vi "Check Home Position Part 2.vi"(8 "error in (no error)":errorcluster, 9 "Amphipods in":refnum<class "Amphipod.lvclass">[](array[class]), 10 "Home":i8, 11 "Position in":cluster{"Row":i8, "Column":i8}) -> (0 "error out":errorcluster, 2 "Position out":cluster{"Row":i8, "Column":i8}[](array[cluster]), 3 "Column":i8)   [LabVIEW 2019, in "23.lvlib" / "Amphipod.lvclass"]
uses:
  Amphipod.lvclass
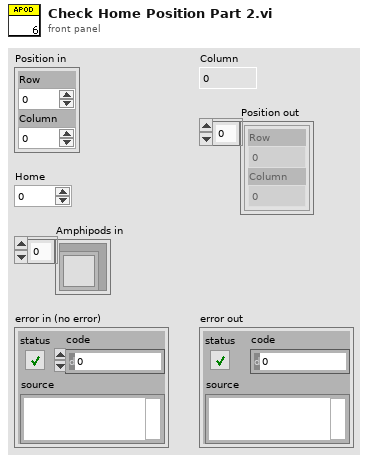
[diagram p1: front panel]
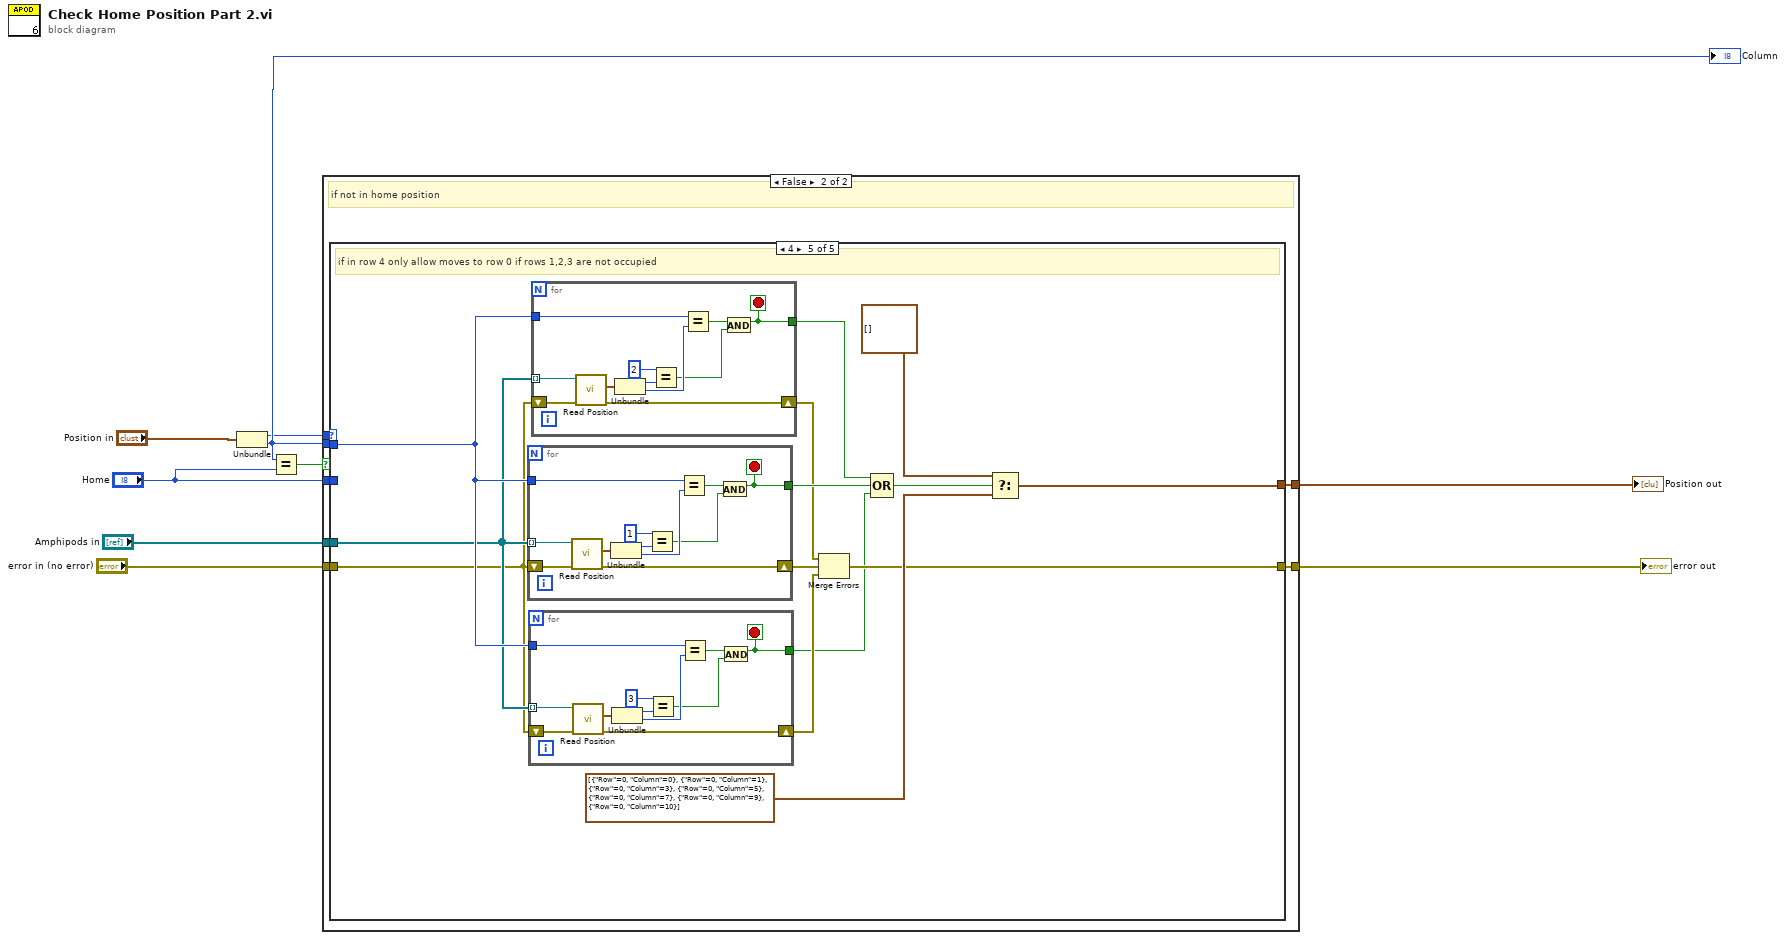
[diagram p0: block diagram]
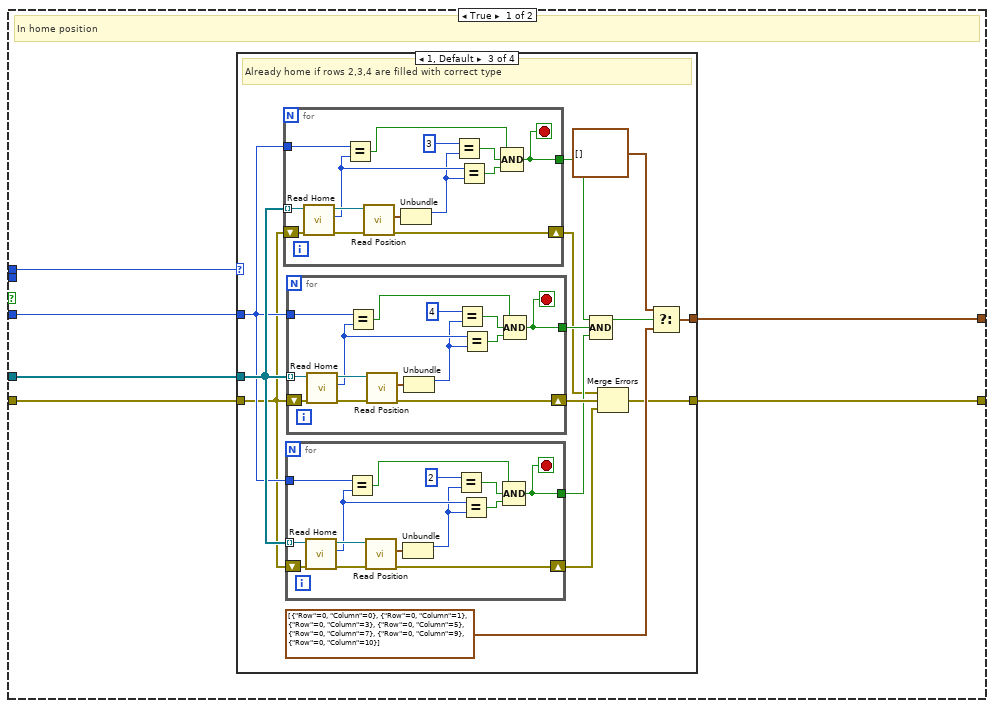
[diagram p2: hidden frame]
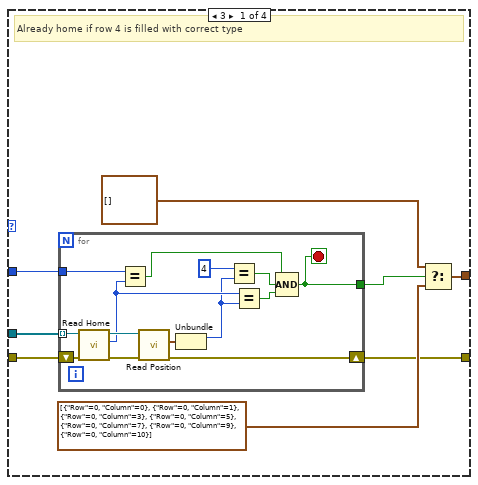
[diagram p3: hidden frame]
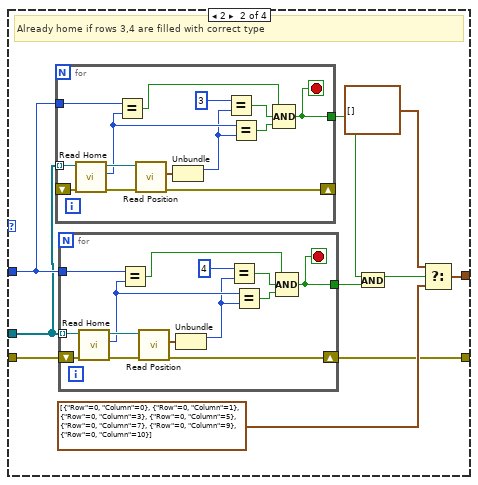
[diagram p4: hidden frame]
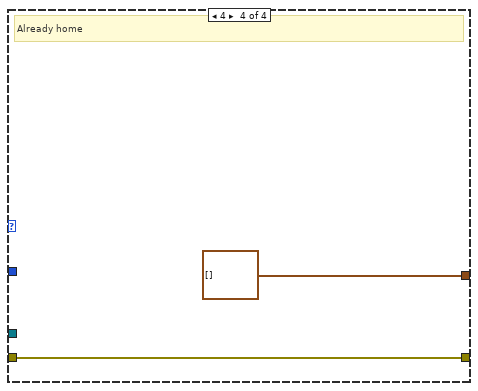
[diagram p5: hidden frame]
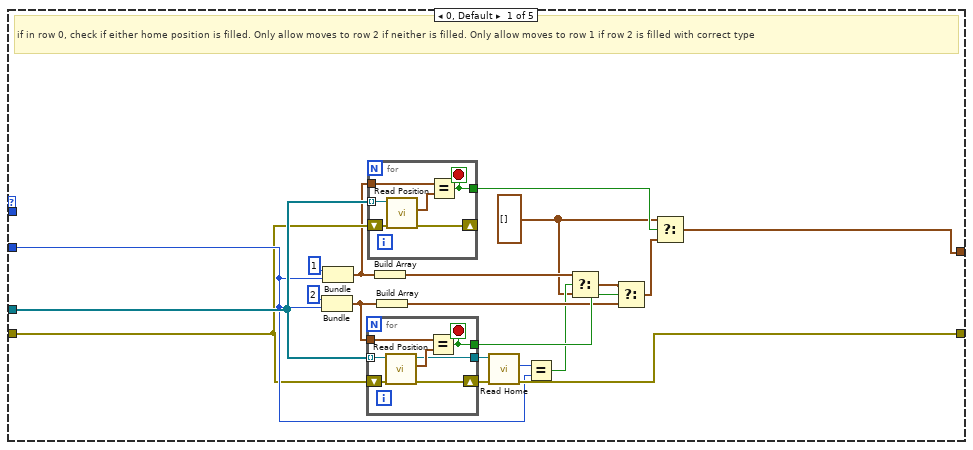
[diagram p6: hidden frame]
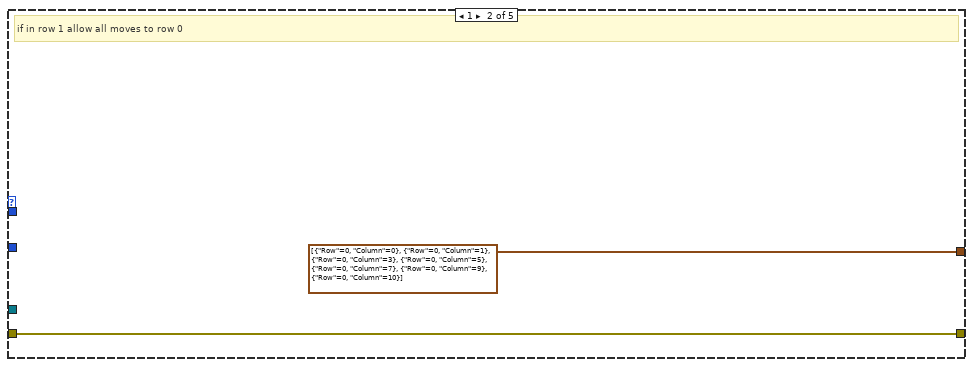
[diagram p7: hidden frame]
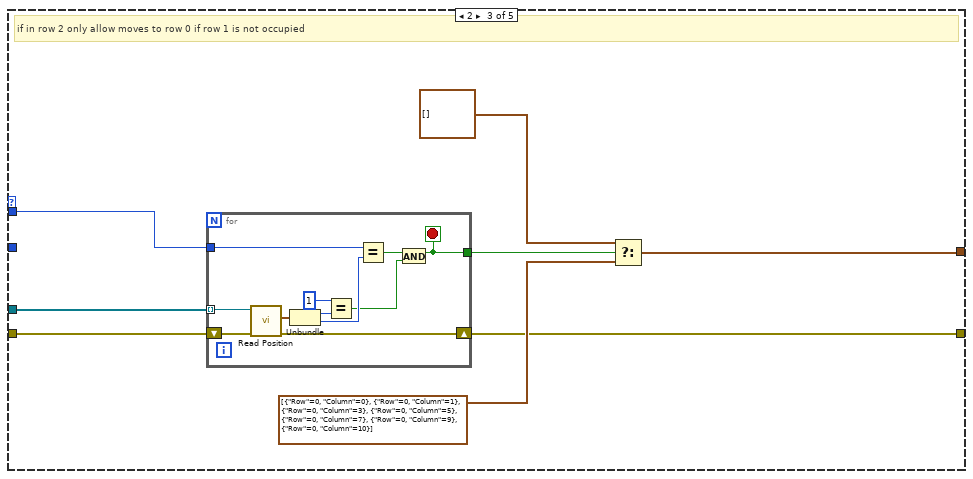
[diagram p8: hidden frame]
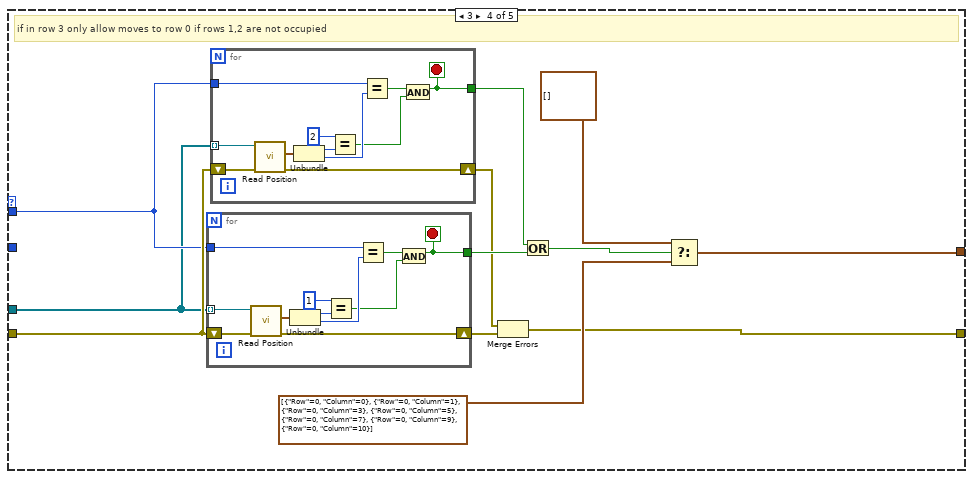
[diagram p9: hidden frame]
diagram:
  n1 = Unbundle("Position in") -> ("Row"=w2:i8, "Column"=w9:i8)
  "Column" <- w9
  n2 = Equal?(x=w9, y="Home") -> (x = y?=w1:bool)
  n3 = case shown="False" w1 {
    tunnel: "Amphipods in" -> [w14 w139]
    tunnel: w2 -> [w15 w140]
    tunnel: "Home" -> [w13 w138]
    tunnel: [w12 w137] -> w5
    tunnel: "error in (no error)" -> [w11 w136]
    tunnel: [w10 w135] -> w8
    tunnel: w9 -> [_ w134]
    frame True {
      # "In home position"
      n4 = case shown="1, Default" w15 {
        tunnel: w14 -> [w23 w40 w82 _]
        tunnel: w13 -> [w17 w41 w81 _]
        tunnel: [w20 w45 w87 cluster{"Row":i8, "Column":i8}[] [] ("t")] -> w12
        tunnel: w11 -> [w19 w44 w76 w132]
        tunnel: [w18 w43 w79 w132] -> w10
        frame 3 {
          # "Already home if row 4 is filled with correct type"
          n5 = for {
            tunnel: w23 -> [w37] mode=indexing
            tunnel: w17 -> [w36]
            shift-right: [w30] -> w18
            shift-left: w19 -> [w35]
            tunnel: [w24] -> w16
            stop <- w24 stop-if-true
            n6 = call-dynamic "Read Home.vi"("error in (no error)"=w35, "Amphipod in"=w37) -> ("error out"=w31:errorcluster, "Home"=w29:i8, "Amphipod out"=w32:refnum<class "Amphipod.lvclass">)  [unwired: 7 in]
            n7 = Equal?(x=w36, y=w29) -> (x = y?=w25:bool)
            n8 = call-dynamic "Read Position.vi"("error in (no error)"=w31, "Amphipod in"=w32) -> ("error out"=w30:errorcluster, "Position"=w34:cluster{"Row":i8, "Column":i8})  [unwired: 7 in, 1 out]
            n9 = Unbundle(w34) -> ("Row"=w28:i8)  [unwired: 1 out]
            n10 = Equal?(x=i8 4, y=w28) -> (x = y?=w27:bool)
            n11 = Equal?(x=w29, y=w28) -> (x = y?=w26:bool)
            n12 = Compound Arithmetic op=AND(w25, w27, w26) -> (w24:bool)
          }
          n13 = Select(t=cluster{"Row":i8, "Column":i8}[] [], s=w16, f=cluster{"Row":i8, "Column":i8}[] [{"Row"=0, "Column"=0}, {"Row"=0, "Column"=1}, {"Row"=0, "Column"=3}, {"Row"=0, "Column"=5}, {"Row"=0, "Column"=7}, {"Row"=0, "Column"=9}, {"Row"=0, "Column"=10}] ("Position")) -> (s? t:f=w20:cluster{"Row":i8, "Column":i8}[])
        }
        frame 2 {
          # "Already home if rows 3,4 are filled with correct type"
          n14 = for {
            tunnel: w40 -> [w61] mode=indexing
            tunnel: w41 -> [w48]
            shift-right: [w55] -> _
            shift-left: _ -> [w60]
            tunnel: [w49] -> w38
            stop <- w49 stop-if-true
            n15 = call-dynamic "Read Home.vi"("error in (no error)"=w60, "Amphipod in"=w61) -> ("error out"=w56:errorcluster, "Home"=w54:i8, "Amphipod out"=w57:refnum<class "Amphipod.lvclass">)  [unwired: 7 in]
            n16 = Equal?(x=w48, y=w54) -> (x = y?=w50:bool)
            n17 = call-dynamic "Read Position.vi"("error in (no error)"=w56, "Amphipod in"=w57) -> ("error out"=w55:errorcluster, "Position"=w59:cluster{"Row":i8, "Column":i8})  [unwired: 7 in, 1 out]
            n18 = Unbundle(w59) -> ("Row"=w53:i8)  [unwired: 1 out]
            n19 = Equal?(x=i8 3, y=w53) -> (x = y?=w52:bool)
            n20 = Equal?(x=w54, y=w53) -> (x = y?=w51:bool)
            n21 = Compound Arithmetic op=AND(w50, w52, w51) -> (w49:bool)
          }
          n22 = for {
            tunnel: w40 -> [w75] mode=indexing
            tunnel: w41 -> [w74]
            shift-right: [w68] -> w43
            shift-left: w44 -> [w73]
            tunnel: [w62] -> w42
            stop <- w62 stop-if-true
            n23 = call-dynamic "Read Home.vi"("error in (no error)"=w73, "Amphipod in"=w75) -> ("error out"=w69:errorcluster, "Home"=w67:i8, "Amphipod out"=w70:refnum<class "Amphipod.lvclass">)  [unwired: 7 in]
            n24 = Equal?(x=w74, y=w67) -> (x = y?=w63:bool)
            n25 = call-dynamic "Read Position.vi"("error in (no error)"=w69, "Amphipod in"=w70) -> ("error out"=w68:errorcluster, "Position"=w72:cluster{"Row":i8, "Column":i8})  [unwired: 7 in, 1 out]
            n26 = Unbundle(w72) -> ("Row"=w66:i8)  [unwired: 1 out]
            n27 = Equal?(x=i8 4, y=w66) -> (x = y?=w65:bool)
            n28 = Equal?(x=w67, y=w66) -> (x = y?=w64:bool)
            n29 = Compound Arithmetic op=AND(w63, w65, w64) -> (w62:bool)
          }
          n30 = And(x=w38, y=w42) -> (x .and. y?=w39:bool)
          n31 = Select(t=cluster{"Row":i8, "Column":i8}[] [], s=w39, f=cluster{"Row":i8, "Column":i8}[] [{"Row"=0, "Column"=0}, {"Row"=0, "Column"=1}, {"Row"=0, "Column"=3}, {"Row"=0, "Column"=5}, {"Row"=0, "Column"=7}, {"Row"=0, "Column"=9}, {"Row"=0, "Column"=10}] ("Position")) -> (s? t:f=w45:cluster{"Row":i8, "Column":i8}[])
        }
        frame 1, Default {
          # "Already home if rows 2,3,4 are filled with correct type"
          n32 = for {
            tunnel: w82 -> [w117] mode=indexing
            tunnel: w81 -> [w104]
            shift-right: [w111] -> w77
            shift-left: w76 -> [w116]
            tunnel: [w105] -> w83
            stop <- w105 stop-if-true
            n33 = call-dynamic "Read Home.vi"("error in (no error)"=w116, "Amphipod in"=w117) -> ("error out"=w112:errorcluster, "Home"=w110:i8, "Amphipod out"=w113:refnum<class "Amphipod.lvclass">)  [unwired: 7 in]
            n34 = Equal?(x=w104, y=w110) -> (x = y?=w106:bool)
            n35 = call-dynamic "Read Position.vi"("error in (no error)"=w112, "Amphipod in"=w113) -> ("error out"=w111:errorcluster, "Position"=w115:cluster{"Row":i8, "Column":i8})  [unwired: 7 in, 1 out]
            n36 = Unbundle(w115) -> ("Row"=w109:i8)  [unwired: 1 out]
            n37 = Equal?(x=i8 3, y=w109) -> (x = y?=w108:bool)
            n38 = Equal?(x=w110, y=w109) -> (x = y?=w107:bool)
            n39 = Compound Arithmetic op=AND(w106, w108, w107) -> (w105:bool)
          }
          n40 = for {
            tunnel: w82 -> [w103] mode=indexing
            tunnel: w81 -> [w102]
            shift-right: [w96] -> w78
            shift-left: w76 -> [w101]
            tunnel: [w90] -> w80
            stop <- w90 stop-if-true
            n41 = call-dynamic "Read Home.vi"("error in (no error)"=w101, "Amphipod in"=w103) -> ("error out"=w97:errorcluster, "Home"=w95:i8, "Amphipod out"=w98:refnum<class "Amphipod.lvclass">)  [unwired: 7 in]
            n42 = Equal?(x=w102, y=w95) -> (x = y?=w91:bool)
            n43 = call-dynamic "Read Position.vi"("error in (no error)"=w97, "Amphipod in"=w98) -> ("error out"=w96:errorcluster, "Position"=w100:cluster{"Row":i8, "Column":i8})  [unwired: 7 in, 1 out]
            n44 = Unbundle(w100) -> ("Row"=w94:i8)  [unwired: 1 out]
            n45 = Equal?(x=i8 2, y=w94) -> (x = y?=w93:bool)
            n46 = Equal?(x=w95, y=w94) -> (x = y?=w92:bool)
            n47 = Compound Arithmetic op=AND(w91, w93, w92) -> (w90:bool)
          }
          n48 = for {
            tunnel: w82 -> [w131] mode=indexing
            tunnel: w81 -> [w130]
            shift-right: [w124] -> w86
            shift-left: w76 -> [w129]
            tunnel: [w118] -> w85
            stop <- w118 stop-if-true
            n49 = call-dynamic "Read Home.vi"("error in (no error)"=w129, "Amphipod in"=w131) -> ("error out"=w125:errorcluster, "Home"=w123:i8, "Amphipod out"=w126:refnum<class "Amphipod.lvclass">)  [unwired: 7 in]
            n50 = Equal?(x=w130, y=w123) -> (x = y?=w119:bool)
            n51 = call-dynamic "Read Position.vi"("error in (no error)"=w125, "Amphipod in"=w126) -> ("error out"=w124:errorcluster, "Position"=w128:cluster{"Row":i8, "Column":i8})  [unwired: 7 in, 1 out]
            n52 = Unbundle(w128) -> ("Row"=w122:i8)  [unwired: 1 out]
            n53 = Equal?(x=i8 4, y=w122) -> (x = y?=w121:bool)
            n54 = Equal?(x=w123, y=w122) -> (x = y?=w120:bool)
            n55 = Compound Arithmetic op=AND(w119, w121, w120) -> (w118:bool)
          }
          n56 = Compound Arithmetic op=AND(w83, w85, w80) -> (w84:bool)
          n57 = Merge Errors(w77, w86, w78) -> (w79:errorcluster)
          n58 = Select(t=cluster{"Row":i8, "Column":i8}[] [], s=w84, f=cluster{"Row":i8, "Column":i8}[] [{"Row"=0, "Column"=0}, {"Row"=0, "Column"=1}, {"Row"=0, "Column"=3}, {"Row"=0, "Column"=5}, {"Row"=0, "Column"=7}, {"Row"=0, "Column"=9}, {"Row"=0, "Column"=10}] ("Position")) -> (s? t:f=w87:cluster{"Row":i8, "Column":i8}[])
        }
        frame 4 {
          # "Already home"
        }
      }
    }
    frame False {
      # "if not in home position"
      n59 = case shown="4" w140 {
        tunnel: w139 -> [w158 _ w183 w199 w232]
        tunnel: w138 -> [w151 _ _ _ _]
        tunnel: [w156 cluster{"Row":i8, "Column":i8}[] [{"Row"=0, "Column"=0}, {"Row"=0, "Column"=1}, {"Row"=0, "Column"=3}, {"Row"=0, "Column"=5}, {"Row"=0, "Column"=7}, {"Row"=0, "Column"=9}, {"Row"=0, "Column"=10}] ("Position") w180 w204 w240] -> w137
        tunnel: w136 -> [w149 w175 w179 w201 w231]
        tunnel: [w153 w175 w177 w196 w235] -> w135
        tunnel: w134 -> [_ _ w176 w200 w233]
        frame 0, Default {
          w141 = cluster{"Row":i8, "Column":i8}[] [] ("t")
          # "if in row 0, check if either home position is filled. Only allow moves to row 2 if neither is filled. Only allow moves to row 1 if row 2 is filled with correct type"
          n60 = Bundle("Row"=i8 2, "Home"=w151) -> (w146:cluster{"Row":i8, "Home":i8})  [unwired: 1 in]
          n61 = Bundle("Row"=i8 1, "Home"=w151) -> (w148:cluster{"Row":i8, "Home":i8})  [unwired: 1 in]
          n62 = for {
            tunnel: w158 -> [w173] mode=indexing
            tunnel: w146 -> [w170]
            shift-right: [w168] -> w154
            shift-left: w149 -> [w172]
            tunnel: [w169] -> w150
            tunnel: [w167] -> w155
            stop <- w169 stop-if-true
            n63 = call-dynamic "Read Position.vi"("error in (no error)"=w172, "Amphipod in"=w173) -> ("error out"=w168:errorcluster, "Position"=w171:cluster{"Row":i8, "Column":i8}, "Amphipod out"=w167:refnum<class "Amphipod.lvclass">)  [unwired: 7 in]
            n64 = Equal?(x=w170, y=w171) -> (x = y?=w169:bool)
          }
          n65 = for {
            tunnel: w158 -> [w161] mode=indexing
            tunnel: w148 -> [w164]
            shift-right: [w163] -> _
            shift-left: w149 -> [w166]
            tunnel: [w162] -> w157
            stop <- w162 stop-if-true
            n66 = call-dynamic "Read Position.vi"("error in (no error)"=w166, "Amphipod in"=w161) -> ("error out"=w163:errorcluster, "Position"=w165:cluster{"Row":i8, "Column":i8})  [unwired: 7 in, 1 out]
            n67 = Equal?(x=w164, y=w165) -> (x = y?=w162:bool)
          }
          n68 = Build Array(w148) -> (w142:cluster{"Row":i8, "Home":i8}[])
          n69 = Build Array(w146) -> (w145:cluster{"Row":i8, "Home":i8}[])
          n70 = call-dynamic "Read Home.vi"("error in (no error)"=w154, "Amphipod in"=w155) -> ("error out"=w153:errorcluster, "Home"=w152:i8)  [unwired: 7 in, 1 out]
          n71 = Equal?(x=w152, y=w151) -> (x = y?=w144:bool)
          n72 = Select(t=w142, s=w144, f=w141) -> (s? t:f=w143:cluster{"Row":i8, "Column":i8}[])
          n73 = Select(t=w143, s=w150, f=w145) -> (s? t:f=w147:cluster{"Row":i8, "Home":i8}[])
          n74 = Select(t=w141, s=w157, f=w147) -> (s? t:f=w156:cluster{"Row":i8, "Home":i8}[])
        }
        frame 1 {
          # "if in row 1 allow all moves to row 0"
        }
        frame 2 {
          # "if in row 2 only allow moves to row 0 if row 1 is not occupied"
          n75 = for {
            tunnel: w183 -> [w193] mode=indexing
            tunnel: w176 -> [w194]
            shift-right: [w189] -> w177
            shift-left: w179 -> [w192]
            tunnel: [w185] -> w178
            stop <- w185 stop-if-true
            n76 = call-dynamic "Read Position.vi"("error in (no error)"=w192, "Amphipod in"=w193) -> ("error out"=w189:errorcluster, "Position"=w191:cluster{"Row":i8, "Column":i8})  [unwired: 7 in, 1 out]
            n77 = Unbundle(w191) -> ("Row"=w187:i8, "Column"=w190:i8)
            n78 = Equal?(x=i8 1, y=w187) -> (x = y?=w184:bool)
            n79 = Equal?(x=w194, y=w190) -> (x = y?=w188:bool)
            n80 = And(x=w188, y=w184) -> (x .and. y?=w185:bool)
          }
          n81 = Select(t=cluster{"Row":i8, "Column":i8}[] [], s=w178, f=cluster{"Row":i8, "Column":i8}[] [{"Row"=0, "Column"=0}, {"Row"=0, "Column"=1}, {"Row"=0, "Column"=3}, {"Row"=0, "Column"=5}, {"Row"=0, "Column"=7}, {"Row"=0, "Column"=9}, {"Row"=0, "Column"=10}] ("Position")) -> (s? t:f=w180:cluster{"Row":i8, "Column":i8}[])
        }
        frame 3 {
          # "if in row 3 only allow moves to row 0 if rows 1,2 are not occupied"
          n82 = for {
            tunnel: w199 -> [w227] mode=indexing
            tunnel: w200 -> [w228]
            shift-right: [w223] -> w202
            shift-left: w201 -> [w226]
            tunnel: [w219] -> w203
            stop <- w219 stop-if-true
            n83 = call-dynamic "Read Position.vi"("error in (no error)"=w226, "Amphipod in"=w227) -> ("error out"=w223:errorcluster, "Position"=w225:cluster{"Row":i8, "Column":i8})  [unwired: 7 in, 1 out]
            n84 = Unbundle(w225) -> ("Row"=w221:i8, "Column"=w224:i8)
            n85 = Equal?(x=i8 1, y=w221) -> (x = y?=w218:bool)
            n86 = Equal?(x=w228, y=w224) -> (x = y?=w222:bool)
            n87 = And(x=w222, y=w218) -> (x .and. y?=w219:bool)
          }
          n88 = for {
            tunnel: w199 -> [w216] mode=indexing
            tunnel: w200 -> [w217]
            shift-right: [w212] -> w195
            shift-left: w201 -> [w215]
            tunnel: [w208] -> w197
            stop <- w208 stop-if-true
            n89 = call-dynamic "Read Position.vi"("error in (no error)"=w215, "Amphipod in"=w216) -> ("error out"=w212:errorcluster, "Position"=w214:cluster{"Row":i8, "Column":i8})  [unwired: 7 in, 1 out]
            n90 = Unbundle(w214) -> ("Row"=w210:i8, "Column"=w213:i8)
            n91 = Equal?(x=i8 2, y=w210) -> (x = y?=w207:bool)
            n92 = Equal?(x=w217, y=w213) -> (x = y?=w211:bool)
            n93 = And(x=w211, y=w207) -> (x .and. y?=w208:bool)
          }
          n94 = Merge Errors(w195, w202) -> (w196:errorcluster)
          n95 = Or(x=w197, y=w203) -> (x .or. y?=w198:bool)
          n96 = Select(t=cluster{"Row":i8, "Column":i8}[] [], s=w198, f=cluster{"Row":i8, "Column":i8}[] [{"Row"=0, "Column"=0}, {"Row"=0, "Column"=1}, {"Row"=0, "Column"=3}, {"Row"=0, "Column"=5}, {"Row"=0, "Column"=7}, {"Row"=0, "Column"=9}, {"Row"=0, "Column"=10}] ("Position")) -> (s? t:f=w204:cluster{"Row":i8, "Column":i8}[])
        }
        frame 4 {
          # "if in row 4 only allow moves to row 0 if rows 1,2,3 are not occupied"
          n97 = for {
            tunnel: w232 -> [w274] mode=indexing
            tunnel: w233 -> [w275]
            shift-right: [w270] -> w238
            shift-left: w231 -> [w273]
            tunnel: [w266] -> w239
            stop <- w266 stop-if-true
            n98 = call-dynamic "Read Position.vi"("error in (no error)"=w273, "Amphipod in"=w274) -> ("error out"=w270:errorcluster, "Position"=w272:cluster{"Row":i8, "Column":i8})  [unwired: 7 in, 1 out]
            n99 = Unbundle(w272) -> ("Row"=w268:i8, "Column"=w271:i8)
            n100 = Equal?(x=i8 1, y=w268) -> (x = y?=w265:bool)
            n101 = Equal?(x=w275, y=w271) -> (x = y?=w269:bool)
            n102 = And(x=w269, y=w265) -> (x .and. y?=w266:bool)
          }
          n103 = for {
            tunnel: w232 -> [w252] mode=indexing
            tunnel: w233 -> [w253]
            shift-right: [w248] -> w230
            shift-left: w231 -> [w251]
            tunnel: [w244] -> w229
            stop <- w244 stop-if-true
            n104 = call-dynamic "Read Position.vi"("error in (no error)"=w251, "Amphipod in"=w252) -> ("error out"=w248:errorcluster, "Position"=w250:cluster{"Row":i8, "Column":i8})  [unwired: 7 in, 1 out]
            n105 = Unbundle(w250) -> ("Row"=w246:i8, "Column"=w249:i8)
            n106 = Equal?(x=i8 3, y=w246) -> (x = y?=w243:bool)
            n107 = Equal?(x=w253, y=w249) -> (x = y?=w247:bool)
            n108 = And(x=w247, y=w243) -> (x .and. y?=w244:bool)
          }
          n109 = for {
            tunnel: w232 -> [w263] mode=indexing
            tunnel: w233 -> [w264]
            shift-right: [w259] -> w234
            shift-left: w231 -> [w262]
            tunnel: [w255] -> w236
            stop <- w255 stop-if-true
            n110 = call-dynamic "Read Position.vi"("error in (no error)"=w262, "Amphipod in"=w263) -> ("error out"=w259:errorcluster, "Position"=w261:cluster{"Row":i8, "Column":i8})  [unwired: 7 in, 1 out]
            n111 = Unbundle(w261) -> ("Row"=w257:i8, "Column"=w260:i8)
            n112 = Equal?(x=i8 2, y=w257) -> (x = y?=w254:bool)
            n113 = Equal?(x=w264, y=w260) -> (x = y?=w258:bool)
            n114 = And(x=w258, y=w254) -> (x .and. y?=w255:bool)
          }
          n115 = Merge Errors(w234, w238, w230) -> (w235:errorcluster)
          n116 = Compound Arithmetic op=OR(w236, w239, w229) -> (w237:bool)
          n117 = Select(t=cluster{"Row":i8, "Column":i8}[] [], s=w237, f=cluster{"Row":i8, "Column":i8}[] [{"Row"=0, "Column"=0}, {"Row"=0, "Column"=1}, {"Row"=0, "Column"=3}, {"Row"=0, "Column"=5}, {"Row"=0, "Column"=7}, {"Row"=0, "Column"=9}, {"Row"=0, "Column"=10}] ("Position")) -> (s? t:f=w240:cluster{"Row":i8, "Column":i8}[])
        }
      }
    }
  }
  "error out" <- w8
  "Position out" <- w5
